vi "Test.vi"() -> ()   [LabVIEW 2015]
uses:
  MJPEG Reader/MJPEG Reader.lvclass
panel:
  in  "Refresh Button":bool
  out "Picture":picture
  in  "Stop Button":bool
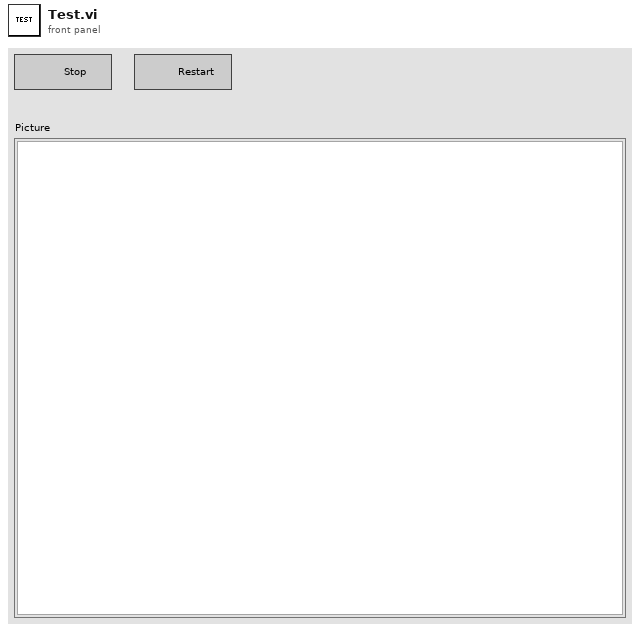
[diagram p1: front panel]
types:
  T1 = cluster{"left":i16, "top":i16, "right":i16, "bottom":i16}
  T2 = typedef "imagedata.ctl" = cluster{"image type":i32, "image depth":i32, "image":u8[], "mask":u8[], "colors":u32[], "Rectangle":cluster{"left":i16, "top":i16, "right":i16, "bottom":i16}}
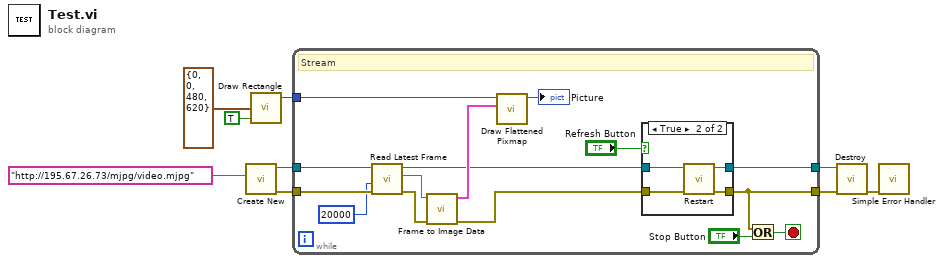
[diagram p0: block diagram]
diagram:
  n1 = call "Create New.vi"("URL"="http://195.67.26.73/mjpg/video.mjpg") -> ("error out"=w8:errorcluster, "MJPEG Reader out"=w9:refnum<data-value>)  [unwired: 9 in]
  n2 = call <vilib>:"Draw Rectangle.vi"("rect"=T1 {"left"=0, "top"=0, "right"=480, "bottom"=620}, "fill?(F)"=TRUE) -> ("new picture"=w2:picture)  [unwired: 7 in]
  n3 = while {
    tunnel: w9 -> [w24]
    tunnel: w8 -> [w23]
    tunnel: [w12] -> w6
    tunnel: [w11] -> w5
    tunnel: w2 -> [w17]
    stop <- w20 stop-if-true
    # "Stream"
    n4 = call "Read Latest Frame.vi"("error in (no error)"=w23, "Read Timeout (ms)"=20000, "MJPEG Reader in"=w24) -> ("error out"=w19:errorcluster, "Frame"=w16:string, "MJPEG Reader out"=w14:refnum<data-value>)  [unwired: 6 in]
    n5 = call "Frame to Image Data.vi"("error in (no error)"=w19, "Frame"=w16) -> ("error out"=w13:errorcluster, "Image Data"=w18:T2)  [unwired: 8 in]
    n6 = call <vilib>:"Draw Flattened Pixmap.vi"("image data"=w18, "picture"=w17) -> ("new picture"=→"Picture":picture)  [unwired: 7 in]
    n7 = case shown="True" "Refresh Button" {
      tunnel: w14 -> [w25 w30]
      tunnel: w13 -> [w26 w29]
      tunnel: [w25 w28] -> w12
      tunnel: [w26 w27] -> w11
      frame False {
      }
      frame True {
        n8 = call "Restart.vi"("error in (no error)"=w29, "MJPEG Reader in"=w30) -> ("error out"=w27:errorcluster, "MJPEG Reader out"=w28:refnum<data-value>)  [unwired: 8 in]
      }
    }
    n9 = Or(x=w11, y="Stop Button") -> (x .or. y?=w20:bool)
  }
  n10 = call "Destroy.vi"("error in (no error)"=w5, "MJPEG Reader in"=w6) -> ("error out"=w4:errorcluster)  [unwired: 9 in]
  n11 = call <vilib>:"Simple Error Handler.vi"("error in (no error)"=w4) -> ()  [unwired: 4 in, 5 out]
